vi "Format String.vi"(1 "String":string) -> (0 "Formated String":string)   [LabVIEW 2018, in "TwinCAT ADS.lvclass"]
uses:
  TwinCAT ADS.lvclass
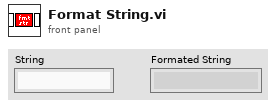
[diagram p1: front panel]
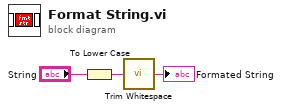
[diagram p0: block diagram]
diagram:
  n1 = To Lower Case(string="String") -> (all lower case string=w3:string)
  n2 = call <vilib>:"Trim Whitespace.vi"("string"=w3) -> ("trimmed string"=→"Formated String":string)  [unwired: 1 in]
